vi "NetworkTable set.vi"   [LabVIEW 2014]
uses:
  Robot Values.vi
  <vilib>/Rock Robotics/Network Tables/SD Write Number.vi
types:
  T1 = cluster{"Lift Encoder Height Right (cm)":dbl, "Lift Encoder Height Left (cm)":dbl, "Right Prox":bool, "Left Prox":bool, "Gyro Angle":dbl, "Gyro anglar rate":dbl}
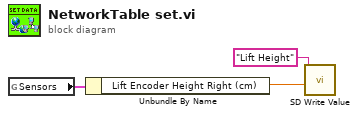
[diagram p0: block diagram]
diagram:
  n1 = global read "Robot Values.vi" "Sensors"() -> (w2:T1)
  n2 = Unbundle By Name(w2) -> ("Lift Encoder Height Right (cm)"=w1:dbl)
  n3 = call-poly <vilib>:"SD Write Value.vi"("Numeric"=w1, "Name"="Lift Height") -> ()  [unwired: 8 in, 2 out]
